vi "mV2MPa.vi"(11 "Volts In":dbl) -> (3 "MPa Out":dbl)   [LabVIEW 2016]
uses:
  <vilib>/Analysis/NI_AALPro.lvlib
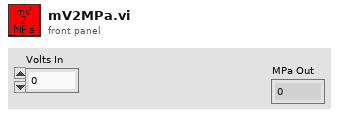
[diagram p1: front panel]
types:
  T1 = cluster{"slope min":dbl, "slope max":dbl, "intercept min":dbl, "intercept max":dbl}
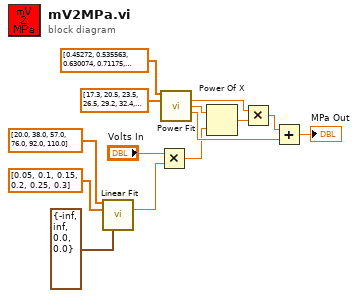
[diagram p0: block diagram]
diagram:
  n1 = call <vilib>:"Linear Fit.vi"("Y"=dbl[] [20.0, 38.0, 57.0, 76.0, 92.0, 110.0], "X"=dbl[] [0.05, 0.1, 0.15, 0.2, 0.25, 0.3], "parameter bounds"=T1 {"slope min"=-inf, "slope max"=inf, "intercept min"=0.0, "intercept max"=0.0}) -> ("slope"=w3:dbl)  [unwired: 8 in, 4 out]
  n2 = Multiply(x="Volts In", y=w3) -> (x*y=w2:dbl)
  n3 = call <vilib>:"Power Fit.vi"("Y"=dbl[] [0.45272, 0.535563, 0.630074, 0.71175, 0.800427, 0.886771, 0.989449, 1.085127, 1.149301, 1.242646, 1.353492, 1.446836, 1.534346, 1.639359, 1.761873, 1.855217, 1.983566, 2.088578, 2.240262, 2.345275], "X"=dbl[] [17.3, 20.5, 23.5, 26.5, 29.2, 32.4, 35.1, 38.0, 41.0, 44.0, 47.2, 49.9, 52.9, 55.9, 58.8, 61.8, 64.6, 67.4, 70.0, 73.0]) -> ("amplitude"=w11:dbl, "power"=w13:dbl, "offset"=w10:dbl)  [unwired: 8 in, 3 out]
  n4 = Power Of X(1:w2, 2:w13) -> (0:w12:dbl)
  n5 = Multiply(x=w11, y=w12) -> (x*y=w9:dbl)
  n6 = Add(x=w9, y=w10) -> (x+y=→"MPa Out":dbl)
